vi "User - Update User Table.vi"(8 "Error In":errorcluster, 9 "Max visible row":i32=7, 10 "User Infor Ref":refnum<vi>, 11 "User Information":string[][](array[string])) -> (0 "Error Out":errorcluster, 3 "User Information Out":T1[](array[typedef]))   [LabVIEW 2020]
uses:
  Control/Cluster - User Information.ctl
  Control/Header - User Management.ctl
panel:
  in  "Access Level":string(combo)="Manager"
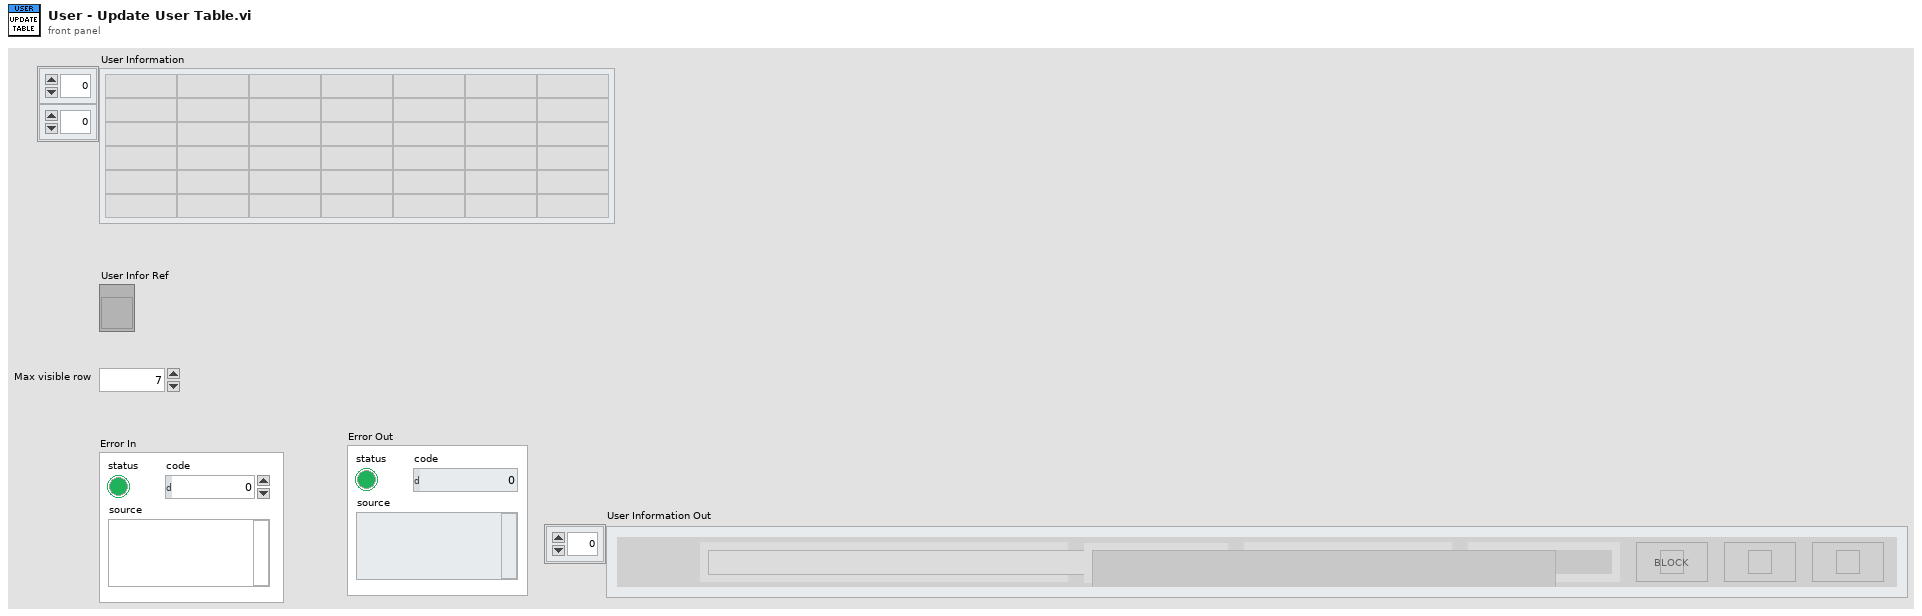
[diagram p1: front panel]
types:
  T1 = typedef "Cluster - User Information.ctl" = cluster{"Access Level":u16, "Name":string, "Staff ID":string, "Username":string, "Password":string, "Configure":bool, "Status":bool, "Remove":bool}
  T2 = typedef "Header - User Management.ctl" = enum16{"Name", "Staff ID", "Username", "Password", "Access Level", "Status", "Access Page"}
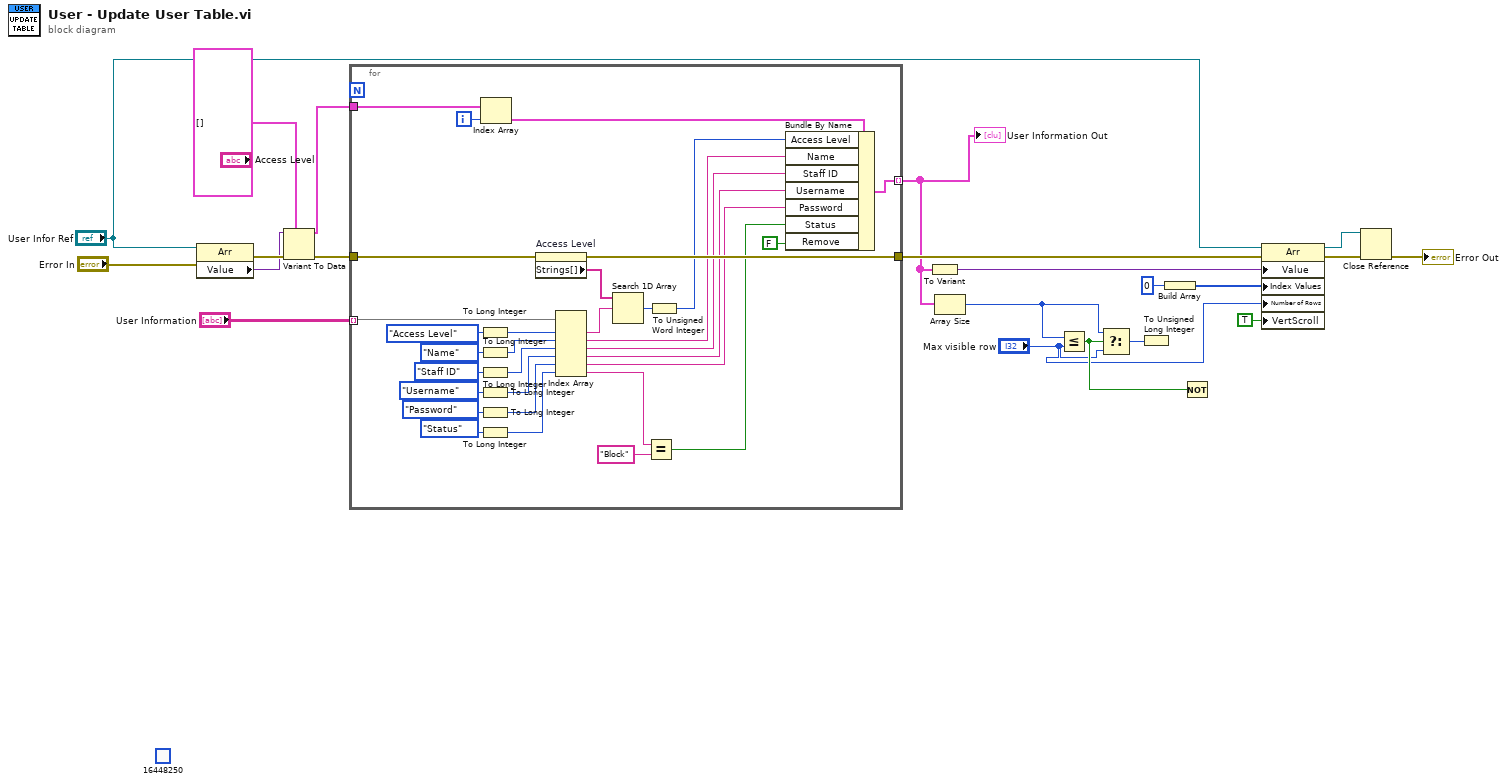
[diagram p0: block diagram]
diagram:
  (unwired) u32 16448250
  n1 = property class="Arr"(reference="User Infor Ref", error in="Error In") -> (error out=w20:errorcluster, "Value"=w14:variant)  [unwired: 1 out]
  n2 = Variant To Data(error in=w20, type=T1[] [] ("Cluster 5"), Variant=w14) -> (data=w13:T1[], error out=w18:errorcluster)
  n3 = for {
    tunnel: "User Information" -> [w50] mode=indexing
    tunnel: w13 -> [w49]
    tunnel: [w45] -> w2 mode=indexing
    tunnel: w18 -> [w51]
    tunnel: [w52] -> w19
    i -> [w43]
    n4 = To Long Integer(number=Header_-_User_Management."Access Level" ("Header - User Management")) -> (32bit integer=w36:i32)
    n5 = To Long Integer(number=Header_-_User_Management."Name" ("Header - User Management")) -> (32bit integer=w35:i32)
    n6 = To Long Integer(number=Header_-_User_Management."Staff ID" ("Header - User Management")) -> (32bit integer=w25:i32)
    n7 = To Long Integer(number=Header_-_User_Management."Username" ("Header - User Management")) -> (32bit integer=w27:i32)
    n8 = To Long Integer(number=Header_-_User_Management."Password" ("Header - User Management")) -> (32bit integer=w28:i32)
    n9 = To Long Integer(number=Header_-_User_Management."Status" ("Header - User Management")) -> (32bit integer=w30:i32)
    n10 = Index Array(array=w49, index=w43) -> (element=w44:T1)
    n11 = property on="Access Level" class="CmbBox"(error in=w51) -> (error out=w52:errorcluster, "Strings[]"=w48:string[])  [unwired: 1 in, 1 out]
    n12 = Index Array(array=w50, index #1=w36, index #2=w35, index #3=w25, index #4=w27, index #5=w28, index #6=w30) -> (element #1=w34:string, element #2=w33:string, element #3=w24:string, element #4=w23:string, element #5=w22:string, element #6=w29:string)
    n13 = Search 1D Array(1D array=w48, element=w34) -> (index of element=w32:i32)  [unwired: 1 in]
    n14 = Equal?(x=w29, y="Block") -> (x = y?=w46:bool)
    n15 = To Unsigned Word Integer(number=w32) -> (unsigned 16bit integer=w31:u16)
    n16 = Bundle By Name(cluster=w44, "Access Level"=w31, "Name"=w33, "Staff ID"=w24, "Username"=w23, "Password"=w22, "Status"=w46, "Remove"=FALSE) -> (w45:T1)
  }
  "User Information Out" <- w2
  n17 = To Variant(anything=w2) -> (Variant=w11:variant)
  n18 = Array Size(array=w2) -> (size(s)=w6:i32)
  n19 = Less Or Equal?(x=w6, y="Max visible row") -> (x <= y?=w4:bool)
  n20 = Select(t=w6, s=w4, f="Max visible row") -> (s? t:f=w5:i32)
  n21 = To Unsigned Long Integer(number=w5) -> ()  [unwired: 1 out]
  n22 = Build Array(u32 0) -> (w8:u32[])
  n23 = Not(x=w4) -> ()  [unwired: 1 out]
  n24 = property class="Arr"(reference="User Infor Ref", error in=w19, "Value"=w11, "Index Values"=w8, "Number of Rows"="Max visible row", "VertScroll"=TRUE ("Vertical Scrollbar Visible")) -> (reference out=w7:refnum<vi>, error out=w17:errorcluster)
  n25 = Close Reference(reference=w7, error in (no error)=w17) -> (error out=→"Error Out":errorcluster)
